vi "ShooterLUT.vi"(11 "Distance from Boiler":dbl) -> (2 "Bottom RPM":dbl, 3 "Top RPM":dbl)   [LabVIEW 2016]
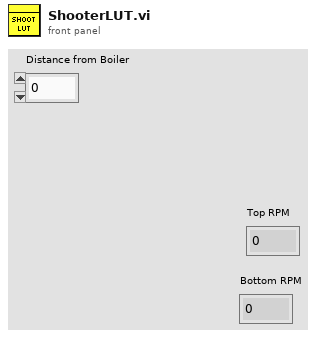
[diagram p1: front panel]
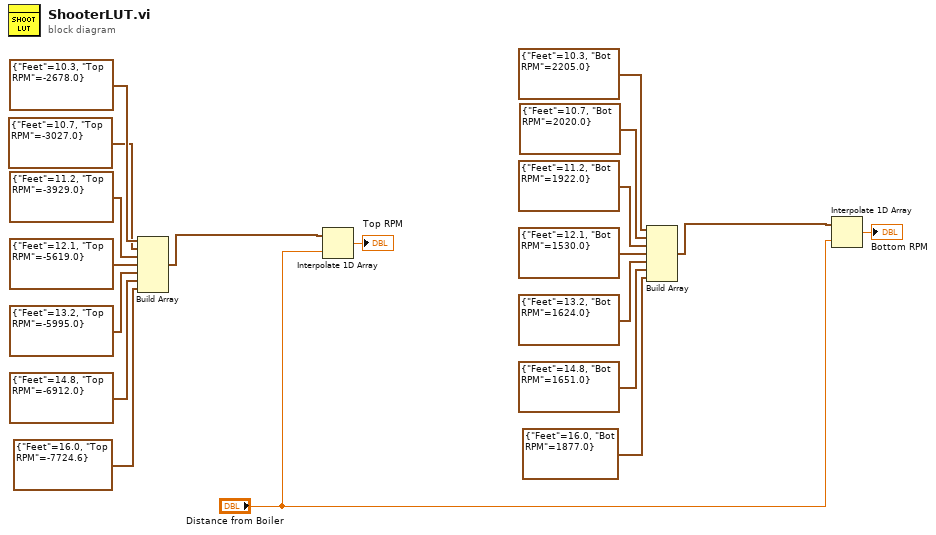
[diagram p0: block diagram]
diagram:
  n1 = Build Array(cluster{"Feet":dbl, "Top RPM":dbl} {"Feet"=10.3, "Top RPM"=-2678.0}, cluster{"Feet":dbl, "Top RPM":dbl} {"Feet"=10.7, "Top RPM"=-3027.0}, cluster{"Feet":dbl, "Top RPM":dbl} {"Feet"=11.2, "Top RPM"=-3929.0}, cluster{"Feet":dbl, "Top RPM":dbl} {"Feet"=12.1, "Top RPM"=-5619.0}, cluster{"Feet":dbl, "Top RPM":dbl} {"Feet"=13.2, "Top RPM"=-5995.0}, cluster{"Feet":dbl, "Top RPM":dbl} {"Feet"=14.8, "Top RPM"=-6912.0}, cluster{"Feet":dbl, "Top RPM":dbl} {"Feet"=16.0, "Top RPM"=-7724.6}) -> (w19:cluster{"Feet":dbl, "Top RPM":dbl}[])
  n2 = Interpolate 1D Array(1:"Distance from Boiler", 2:w19) -> (0:→"Top RPM":dbl)
  n3 = Build Array(cluster{"Feet":dbl, "Bot RPM":dbl} {"Feet"=10.3, "Bot RPM"=2205.0}, cluster{"Feet":dbl, "Bot RPM":dbl} {"Feet"=10.7, "Bot RPM"=2020.0}, cluster{"Feet":dbl, "Bot RPM":dbl} {"Feet"=11.2, "Bot RPM"=1922.0}, cluster{"Feet":dbl, "Bot RPM":dbl} {"Feet"=12.1, "Bot RPM"=1530.0}, cluster{"Feet":dbl, "Bot RPM":dbl} {"Feet"=13.2, "Bot RPM"=1624.0}, cluster{"Feet":dbl, "Bot RPM":dbl} {"Feet"=14.8, "Bot RPM"=1651.0}, cluster{"Feet":dbl, "Bot RPM":dbl} {"Feet"=16.0, "Bot RPM"=1877.0}) -> (w6:cluster{"Feet":dbl, "Bot RPM":dbl}[])
  n4 = Interpolate 1D Array(1:"Distance from Boiler", 2:w6) -> (0:→"Bottom RPM":dbl)
